vi "2 - Global variable.vi"() -> ()   [LabVIEW 2015]
uses:
  My Globals.vi
panel:
  in  "stop":bool
  out "Chart 3":i32(graph)
  out "Chart 2":dbl(graph)
  out "Chart 1":dbl(graph)
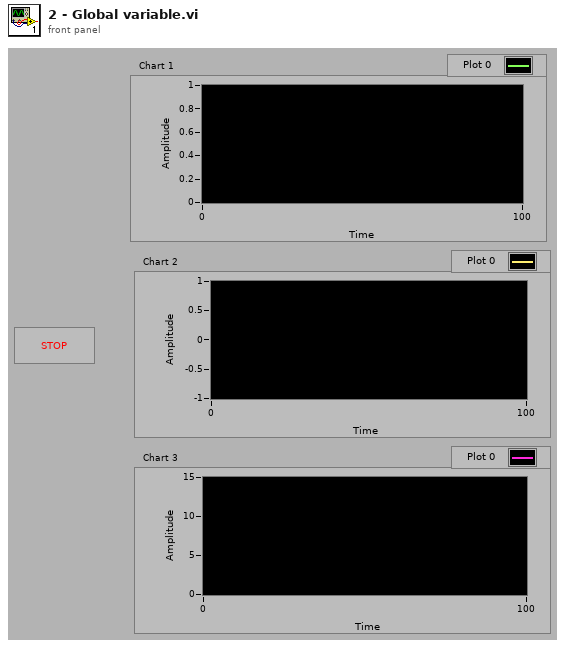
[diagram p1: front panel]
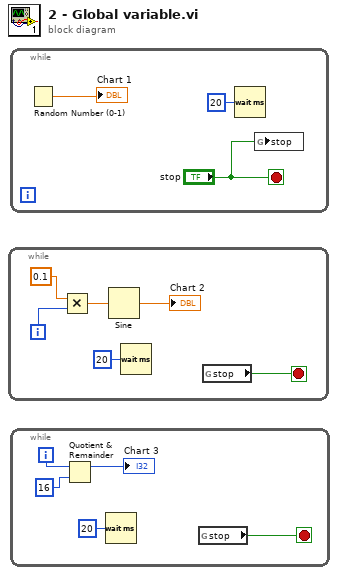
[diagram p0: block diagram]
diagram:
  n1 = while {
    i -> [w4]
    stop <- w1 stop-if-true
    n2 = Multiply(x=0.1, y=w4) -> (x*y=w3:dbl)
    n3 = Sine(x=w3) -> (sin(x)=→"Chart 2":dbl)
    n4 = Wait (ms)(milliseconds to wait=u32 20) -> ()  [unwired: 1 out]
    n5 = global read "My Globals.vi" "stop"() -> (w1:bool)
  }
  n6 = while {
    stop <- "stop" stop-if-true
    n7 = Random Number (0-1)() -> (number: 0 to 1=→"Chart 1":dbl)
    n8 = Wait (ms)(milliseconds to wait=u32 20) -> ()  [unwired: 1 out]
    n9 = global write "My Globals.vi" "stop"("stop") -> ()
  }
  n10 = while {
    i -> [w13]
    stop <- w10 stop-if-true
    n11 = Quotient & Remainder(x=w13, y=16) -> (x-y*floor(x/y)=→"Chart 3":i32)  [unwired: 1 out]
    n12 = Wait (ms)(milliseconds to wait=u32 20) -> ()  [unwired: 1 out]
    n13 = global read "My Globals.vi" "stop"() -> (w10:bool)
  }
